vi "DS写数组数据.vi"() -> ()   [LabVIEW 2010]
uses:
  <vilib>/Analysis/NI_AALBase.lvlib
panel:
  in  "幅值":dbl(slide)=1.0 scale=0.0..10.0
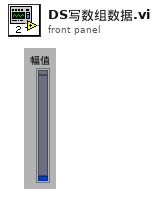
[diagram p1: front panel]
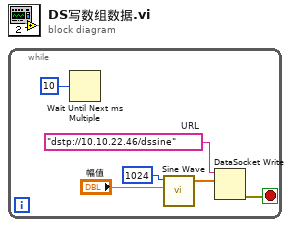
[diagram p0: block diagram]
diagram:
  n1 = while {
    stop <- w5 stop-if-true
    w6 = "dstp://10.10.22.46/dssine"  # URL
    n2 = Wait Until Next ms Multiple(millisecond multiple=u32 10) -> ()  [unwired: 1 out]
    n3 = call <vilib>:"Sine Wave.vi"("samples"=1024, "amplitude"="幅值") -> ("sine wave"=w3:dbl[])  [unwired: 3 in, 2 out]
    n4 = DataSocket Write(10:w3, 11:w6) -> (0:w5:errorcluster)  [unwired: 2 in, 2 out]
  }
